vi "facade.vi"(0 "Data In":T7, 2 "Display State In":T3={"keyboard ref"=refnum, "mouse ref"=refnum, "control refs"={"check mouse"=refnum}, "settings"={"key"=enum."RIGHT", "increment"=0.0}}, 3 "Container State":T6) -> (6 "Data Out":T7, 7 "Display State Out":T3={"keyboard ref"=refnum, "mouse ref"=refnum, "control refs"={"check mouse"=refnum}, "settings"={"key"=enum."RIGHT", "increment"=0.0}}, 8 "Action":T2)   [LabVIEW 2010, in "XMouseSlider.xctl"]
uses:
  XMouseSlider.xctl
  data.ctl
  <vilib>/_xctls/Container State.ctl
  state.ctl
  control_refs_cluster.ctl
  settings_cluster.ctl
  <vilib>/_xctls/Action.ctl
  <vilib>/Utility/inputDevices.llb/mouseAcquire.vi
  <vilib>/Utility/inputDevices.llb/keyboardAcquire.vi
  <vilib>/Utility/inputDevices.llb/closeMouse.vi
  <vilib>/Utility/inputDevices.llb/closeKeyboard.vi
  <vilib>/_xctls/XControlSupport.lvlib
panel:
  in  "?":enum32{"    ", "Settings"}(tab)
  in  "Slide":dbl(slide) scale=0.0..10.0
  in  "increment":dbl
  in  "key":T1(ring)=enum."RIGHT"
  out "check mouse":bool
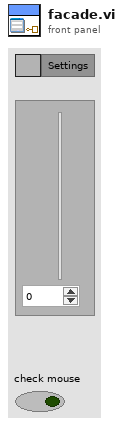
[diagram p1: front panel]
types:
  T1 = enum16{"0", "1", "2", "3", "4", "5", "6", "7", "8", "9", "A", "B", "C", "D", "E", "F", "G", "H", "I", "J", "K", "L", "M", "N", "O", "P", "Q", "R", "S", "T", "U", "V", "W", "X", "Y", "Z", "F1", "F2", "F3", "F4", "F5", "F6", "F7", "F8", "F9", "F10", "F11", "F12", "F13", "F14", "F15", "ADD", "BACK", "BACKSLASH", "CAPITAL", "COMMA", "DECIMAL", "DELETE", "DIVIDE", "DOWN", "END", "EQUALS", "ESCAPE", "GRAVE (`)", "HOME", "INSERT", "LBRACKET", "LCONTROL", "LEFT", "L ALT", "LSHIFT", "LWIN", "MINUS", "MULTIPLY", "NEXT", "NUMLOCK", "NUMPAD_0", "NUMPAD_1", "NUMPAD_2", "NUMPAD_3", "NUMPAD_4", "NUMPAD_5", "NUMPAD_6", "NUMPAD_7", "NUMPAD_8", "NUMPAD_9", "PAUSE", "PERIOD", "PRIOR (PG UP)", "RBRACKET", "RCONTROL", "RETURN", "RIGHT", "R ALT", "RSHIFT", "RWIN", "SCROLL", "SEMICOLON", "SLASH", "SPACE", "SUBTRACT", "TAB", "UP", "ENTER (num pad)", "' (quote)"}
  T2 = typedef "XControlSupport.lvlib/Action.ctl" = cluster{"Data Changed?":bool, "State Changed?":bool, "Action Name":string}
  T3 = typedef "XMouseSlider.xctl/state.ctl" = cluster{"keyboard ref":refnum<k1>, "mouse ref":refnum<k1>, "control refs":T4, "settings":T5}
  T4 = typedef "XMouseSlider.xctl/control_refs_cluster.ctl" = cluster{"check mouse":refnum<vi>}
  T5 = typedef "XMouseSlider.xctl/settings_cluster.ctl" = cluster{"key":enum16{"0", "1", "2", "3", "4", "5", "6", "7", "8", "9", "A", "B", "C", "D", "E", "F", "G", "H", "I", "J", "K", "L", "M", "N", "O", "P", "Q", "R", "S", "T", "U", "V", "W", "X", "Y", "Z", "F1", "F2", "F3", "F4", "F5", "F6", "F7", "F8", "F9", "F10", "F11", "F12", "F13", "F14", "F15", "ADD", "BACK", "BACKSLASH", "CAPITAL", "COMMA", "DECIMAL", "DELETE", "DIVIDE", "DOWN", "END", "EQUALS", "ESCAPE", "GRAVE (`)", "HOME", "INSERT", "LBRACKET", "LCONTROL", "LEFT", "L ALT", "LSHIFT", "LWIN", "MINUS", "MULTIPLY", "NEXT", "NUMLOCK", "NUMPAD_0", "NUMPAD_1", "NUMPAD_2", "NUMPAD_3", "NUMPAD_4", "NUMPAD_5", "NUMPAD_6", "NUMPAD_7", "NUMPAD_8", "NUMPAD_9", "PAUSE", "PERIOD", "PRIOR (PG UP)", "RBRACKET", "RCONTROL", "RETURN", "RIGHT", "R ALT", "RSHIFT", "RWIN", "SCROLL", "SEMICOLON", "SLASH", "SPACE", "SUBTRACT", "TAB", "UP", "ENTER (num pad)", "' (quote)"}, "increment":dbl}
  T6 = typedef "XControlSupport.lvlib/Container State.ctl" = cluster{"Indicator?":bool, "Run Mode?":bool, " Refnum":refnum<vi>}
  T7 = typedef "XMouseSlider.xctl/data.ctl" = dbl
  T8 = cluster{"Horizontal":i32, "Vertical":i32, "Scrolling":i32}
  T9 = enum16{"0", "1", "2", "3", "4", "5", "6", "7", "8", "9", "A", "B", "C", "D", "E", "F", "G", "H", "I", "J", "K", "L", "M", "N", "O", "P", "Q", "R", "S", "T", "U", "V", "W", "X", "Y", "Z", "F1", "F2", "F3", "F4", "F5", "F6", "F7", "F8", "F9", "F10", "F11", "F12", "F13", "F14", "F15", "ADD", "BACK", "BACKSLASH", "CAPITAL", "COMMA", "DECIMAL", "DELETE", "DIVIDE", "DOWN", "END", "EQUALS", "ESCAPE", "GRAVE (`)", "HOME", "INSERT", "LBRACKET", "LCONTROL", "LEFT", "L ALT", "LSHIFT", "LWIN", "MINUS", "MULTIPLY", "NEXT", "NUMLOCK", "NUMPAD_0", "NUMPAD_1", "NUMPAD_2", "NUMPAD_3", "NUMPAD_4", "NUMPAD_5", "NUMPAD_6", "NUMPAD_7", "NUMPAD_8", "NUMPAD_9", "PAUSE", "PERIOD", "PRIOR (PG UP)", "RBRACKET", "RCONTROL", "RETURN", "RIGHT", "R ALT", "RSHIFT", "RWIN", "SCROLL", "SEMICOLON", "SLASH", "SPACE", "SUBTRACT", "TAB", "UP", "ENTER (num pad)", "' (quote)"}[]
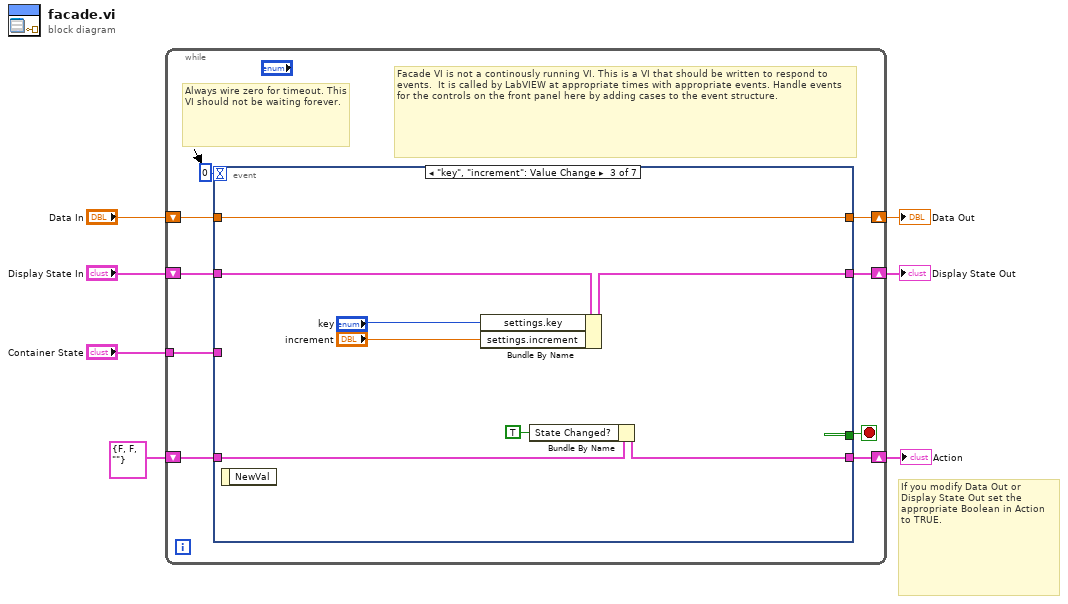
[diagram p0: block diagram]
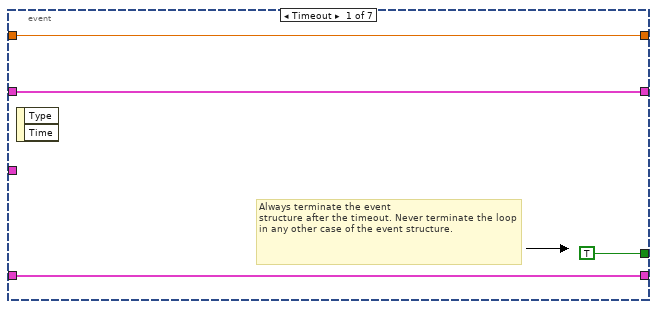
[diagram p2: hidden frame]
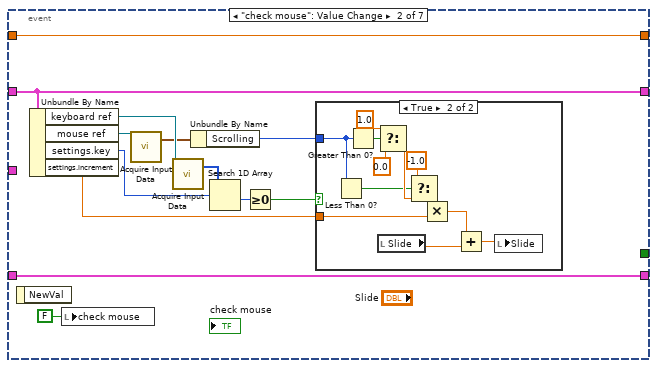
[diagram p3: hidden frame]
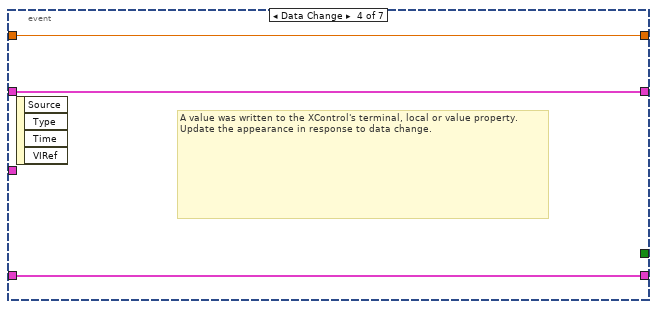
[diagram p5: hidden frame]
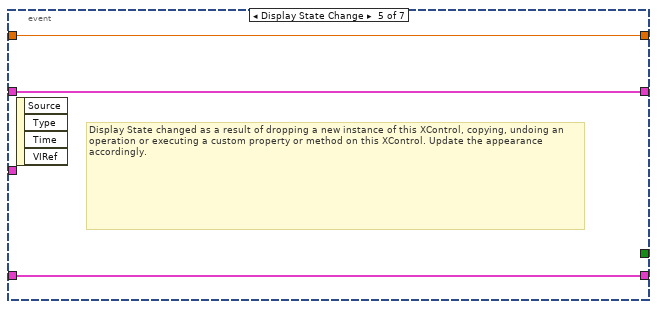
[diagram p6: hidden frame]
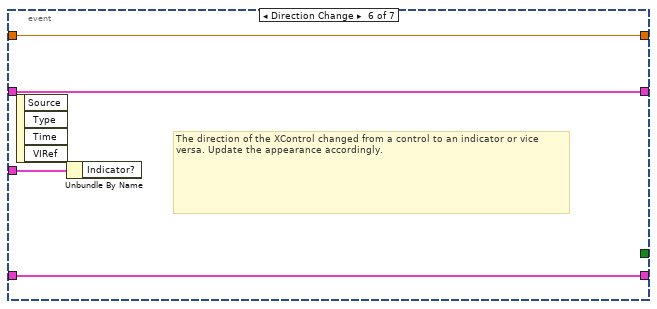
[diagram p7: hidden frame]
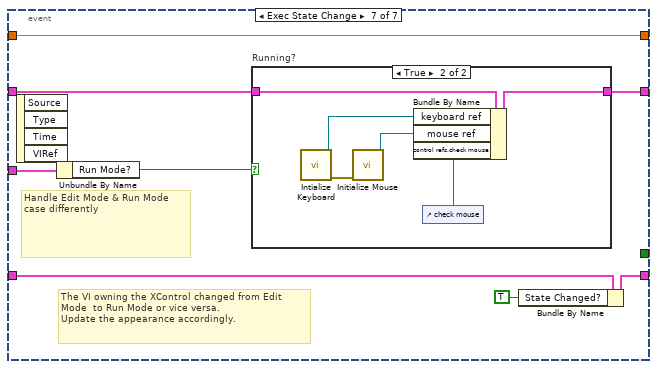
[diagram p8: hidden frame]
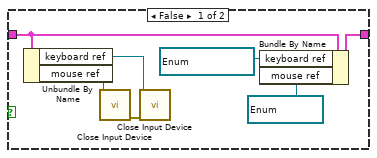
[diagram p9: hidden frame]
diagram:
  # "If you modify Data Out or\nDisplay State Out set the\nappropriate Boolean in Action\nto TRUE."
  n1 = while {
    shift-right: [w15] -> w4
    shift-left: "Display State In" -> [w16]
    tunnel: "Container State" -> [w12]
    shift-right: [w10] -> w7
    shift-left: "Data In" -> [w11]
    shift-right: [w8] -> w2
    shift-left: T2 {"Data Changed?"=FALSE, "State Changed?"=FALSE, "Action Name"=""} ("Action") -> [w9]
    stop <- w14 stop-if-true
    # "Facade VI is not a continously running VI. This is a VI that should be written to respond to events.  It is called by LabVIEW at appropriate times with appropriate events. Handle events for the controls on the front panel here by adding cases to the event structure."
    # "Always wire zero for timeout. This\nVI should not be waiting forever."
    n2 = event shown="[2] \"key\", \"increment\": Value Change" {
      selector: _ -> [_ _ _ _ _ _ _]
      dyn-events: _ -> [_ _ _ _ _ _ _]
      timeout: 0 -> [_ _ _ _ _ _ _]
      tunnel: w16 -> [w18 w30 w52 w55 w59 w62 w69]
      tunnel: [w18 w30 w51 w55 w59 w62 w68] -> w15
      tunnel: [TRUE _ _ _ _ _ _] -> w14
      tunnel: w12 -> [_ _ _ _ _ w63 w71]
      tunnel: w11 -> [w17 w32 w53 w56 w58 w61 w70]
      tunnel: [w17 w32 w53 w56 w58 w61 w70] -> w10
      tunnel: [w19 w31 w46 w54 w57 w60 w64] -> w8
      tunnel: w9 -> [w19 w31 w47 w54 w57 w60 w65]
      event Timeout {
        # "Always terminate the event\nstructure after the timeout. Never terminate the loop in any other case of the event structure."
        n3 = event-data() -> ()  [unwired: 1 in, 2 out]
      }
      event "check mouse": Value Change {
        n4 = event-data() -> ()  [unwired: 1 in, 1 out]
        n5 = Unbundle By Name(w30) -> ("keyboard ref"=w28:refnum<k1>, "mouse ref"=w29:refnum<k1>, "settings.key"=w22:T1, "settings.increment"=w21:dbl)
        n6 = local write "check mouse"(FALSE ("check mouse")) -> ()
        n7 = call-poly <vilib>:"Acquire Input Data.vi"("device ID"=w29) -> ("axis info"=w26:T8)  [unwired: 15 in, 3 out]
        n8 = call-poly <vilib>:"Acquire Input Data.vi"("device ID"=w28) -> ("keys pressed"=w27:T9)  [unwired: 16 in, 2 out]
        n9 = Unbundle By Name(w26) -> ("Scrolling"=w25:i32)
        n10 = Search 1D Array(1D array=w27, element=w22) -> (index of element=w24:i32)  [unwired: 1 in]
        n11 = Greater Or Equal To 0?(x=w24) -> (x >= 0?=w23:bool)
        n12 = case shown="True" w23 {
          tunnel: w25 -> [_ w42]
          tunnel: w21 -> [_ w34]
          frame False {
          }
          frame True {
            n13 = Less Than 0?(x=w42) -> (x < 0?=w40:bool)
            n14 = Greater Than 0?(x=w42) -> (x > 0?=w45:bool)
            n15 = Select(t=1.0, s=w45, f=0.0 ("t")) -> (s? t:f=w41:dbl)
            n16 = local read "Slide"() -> (w35:dbl)
            n17 = Select(t=-1.0, s=w40, f=w41) -> (s? t:f=w38:dbl)
            n18 = Multiply(x=w38, y=w34) -> (x*y=w37:dbl)
            n19 = Add(x=w37, y=w35) -> (x+y=w36:dbl)
            n20 = local write "Slide"(w36) -> ()
          }
        }
      }
      event "key", "increment": Value Change {
        n21 = event-data() -> ()  [unwired: 1 in, 1 out]
        n22 = Bundle By Name(cluster=w52, "settings.key"="key", "settings.increment"="increment") -> (w51:T3)
        n23 = Bundle By Name(cluster=w47, "State Changed?"=TRUE) -> (w46:T2)
      }
      event Data Change {
        # "A value was written to the XControl's terminal, local or value property.\nUpdate the appearance in response to data change."
        n24 = event-data() -> ()  [unwired: 1 in, 4 out]
      }
      event Display State Change {
        # "Display State changed as a result of dropping a new instance of this XControl, copying, undoing an operation or executing a custom property or method on this XControl. Update the appearance accordingly."
        n25 = event-data() -> ()  [unwired: 1 in, 4 out]
      }
      event Direction Change {
        # "The direction of the XControl changed from a control to an indicator or vice versa. Update the appearance accordingly."
        n26 = event-data() -> ()  [unwired: 1 in, 4 out]
        n27 = Unbundle By Name(w63) -> ()  [unwired: 1 out]
      }
      event Exec State Change {
        # "The VI owning the XControl changed from Edit Mode  to Run Mode or vice versa.\nUpdate the appearance accordingly."
        # "Handle Edit Mode & Run Mode\ncase differently"
        n28 = event-data() -> ()  [unwired: 1 in, 4 out]
        n29 = Unbundle By Name(w71) -> ("Run Mode?"=w67:bool)
        n30 = case "Running?" shown="True" w67 {
          tunnel: w69 -> [w75 w81]
          tunnel: [w72 w80] -> w68
          frame False {
            w73 = refnum<k1> refnum items=["MOUSE"] ("mouse ref")
            w74 = refnum<k1> refnum items=["KEYBOARD"] ("keyboard ref")
            n31 = Unbundle By Name(w75) -> ("keyboard ref"=w77:refnum<k1>, "mouse ref"=w78:refnum<k1>)
            n32 = call-poly <vilib>:"Close Input Device.vi"("device ID"=w78) -> ("error out"=w76:errorcluster)  [unwired: 9 in]
            n33 = call-poly <vilib>:"Close Input Device.vi"("error in (no error)"=w76, "device ID"=w77) -> ()  [unwired: 8 in, 1 out]
            n34 = Bundle By Name(cluster=w75, "keyboard ref"=w74, "mouse ref"=w73) -> (w72:T3)
          }
          frame True {
            n35 = call <vilib>:"Intialize Keyboard.vi"() -> ("error out"=w84:errorcluster, "device ID"=w83:refnum<k1>)  [unwired: 10 in]
            n36 = call <vilib>:"Initialize Mouse.vi"("error in (no error)"=w84) -> ("device ID"=w82:refnum<k1>)  [unwired: 9 in, 1 out]
            n37 = control-ref of="check mouse"() -> (w79:refnum<vi>)
            n38 = Bundle By Name(cluster=w81, "keyboard ref"=w83, "mouse ref"=w82, "control refs.check mouse"=w79) -> (w80:T3)
          }
        }
        n39 = Bundle By Name(cluster=w65, "State Changed?"=TRUE) -> (w64:T2)
      }
    }
  }
  "Display State Out" <- w4
  "Data Out" <- w7
  "Action" <- w2
